vi "_PC_Daemon_System.vi"(7 "GetRef? ( F )":bool, 8 "error in (no error)":errorcluster) -> (0 "error out":errorcluster, 2 "Instrument Parmeter":T1)   [LabVIEW 2018]
uses:
  <vilib>/event_ctls.llb/eventvkey.ctl
  PublicSubVI/Class/QMH/QMH.lvclass
panel:
  in  "Config Tab":enum32{"RT Status", "Vacuum", "High Voltage"}(tab)
  out "Time":timestamp
  out "Wfm occupied":string
  out "Firmware Version":string="None"
  out "RT Resource":cluster{timestamp[], dbl[]}[](graph)
  out "Turbo speed":cluster{timestamp, "Double":dbl}[](graph)
  out "Turbo power":cluster{timestamp, "Double":dbl}[](graph)
  out "Pressure chart":cluster{timestamp, "Double":dbl}[](graph)
  out "Turbo pump status":string
  out "Voltage":cluster{timestamp[], dbl[]}[](graph)
  out "break":bool
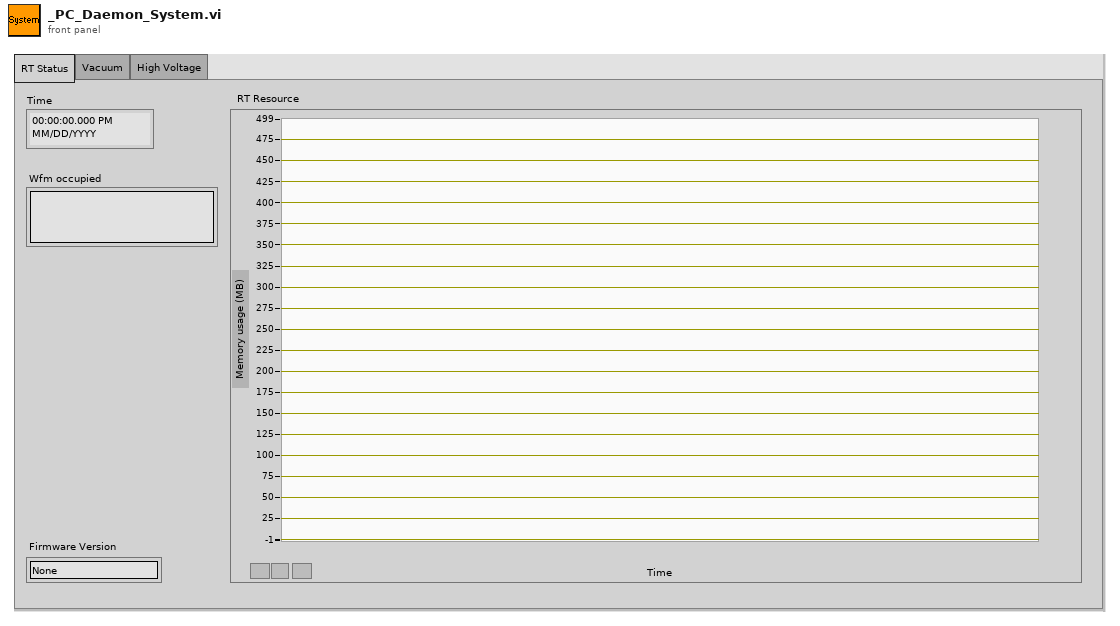
[diagram p1: front panel]
types:
  T1 = cluster{"Pressure chart":refnum<vi>, "Turbo pump status":refnum<vi>, "Turbo speed":refnum<vi>, "Turbo power":refnum<vi>, "RT Resource":refnum<vi>, "Pressure realtime":refnum<vi>, "Voltage":refnum<vi>, "Pressure string":refnum<vi>}
  T2 = typedef "eventvkey.ctl" = enum16{"ASCII", "Enter", "Return", "Shift", "Ctrl", "Alt", "Cmd", "Opt", "Caps", "NumLock", "Clear", "Break", "Up", "Down", "Left", "Right", "Insert", "Delete", "Home", "End", "PageUp", "PageDown", "Escape", "Help", "Pause", "ScrollLock", "F1", "F2", "F3", "F4", "F5", "F6", "F7", "F8", "F9", "F10", "F11", "F12", "F13", "F14", "F15", "F16", "F17", "F18", "F19", "F20", "F21", "F22", "F23", "F24", "Play", "VolumeUp", "VolumeDown", "Mute", "Two Byte Char"}
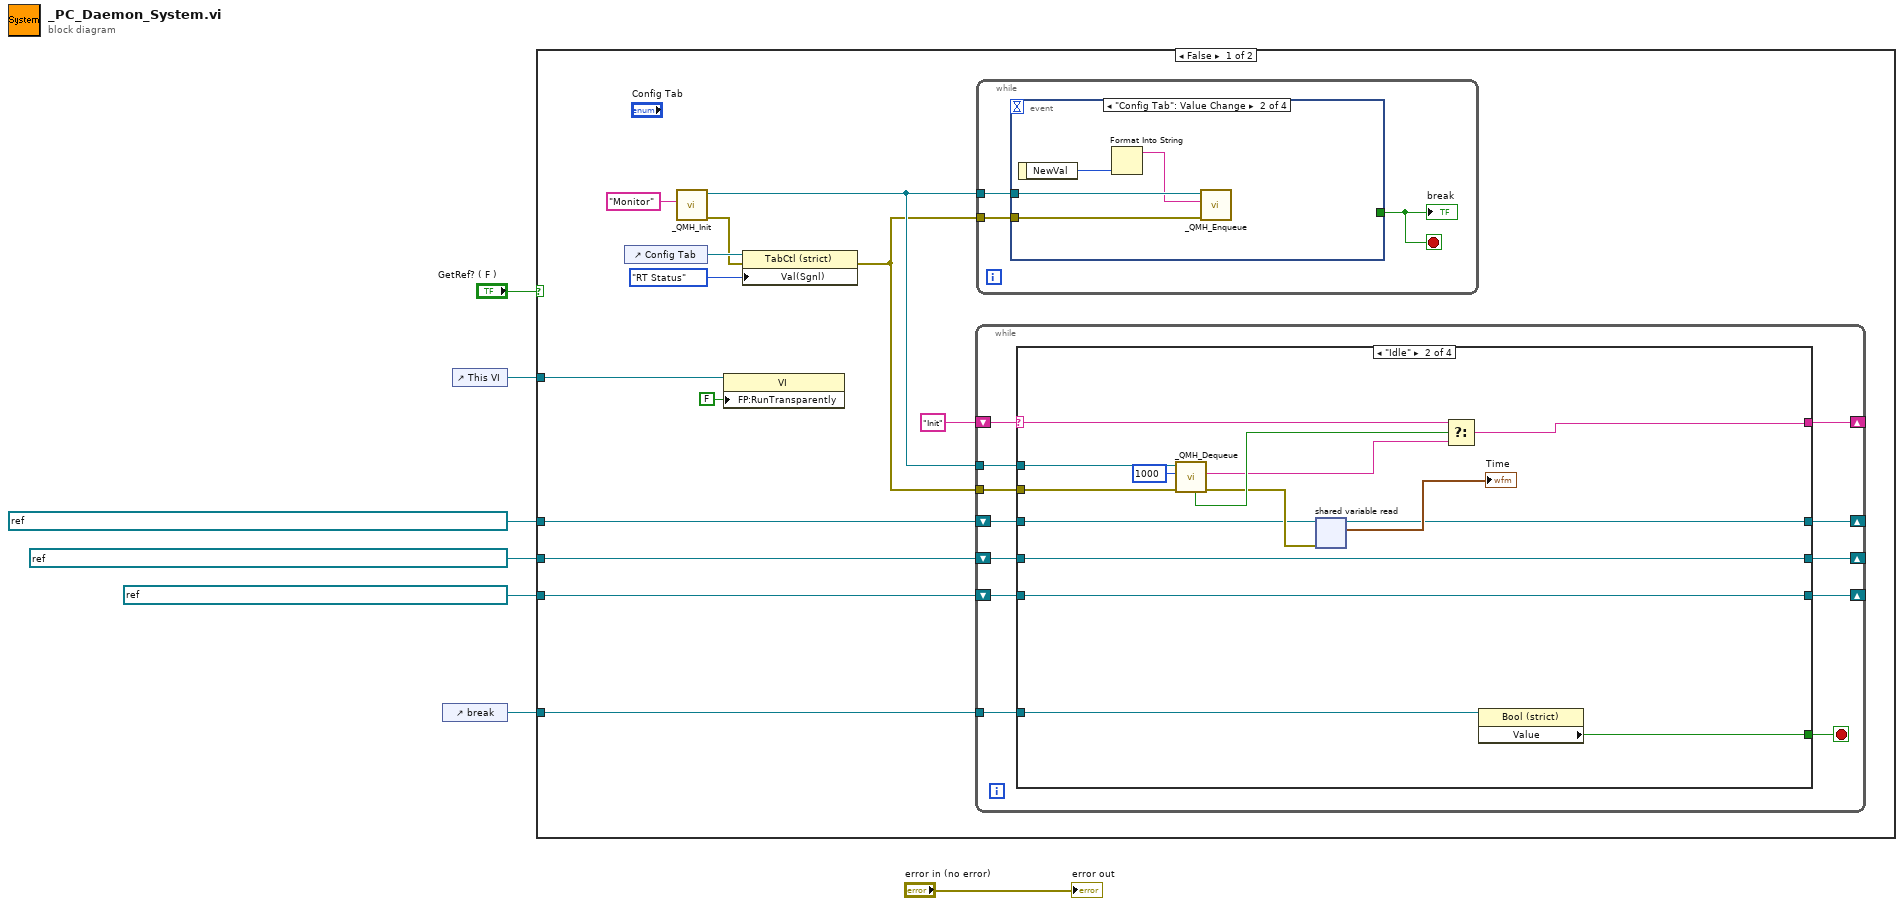
[diagram p0: block diagram]
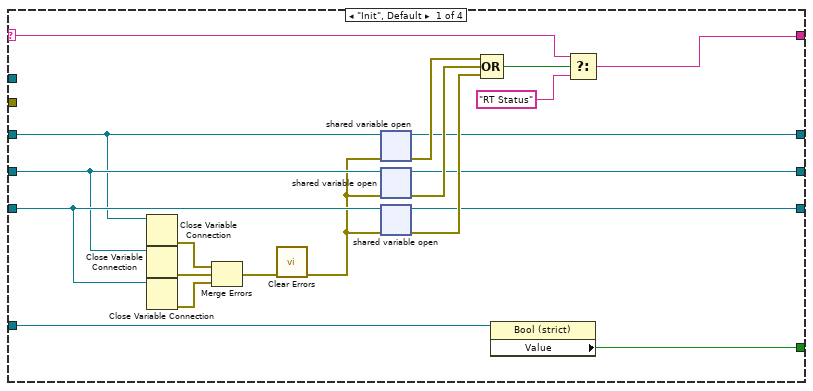
[diagram p2: hidden frame]
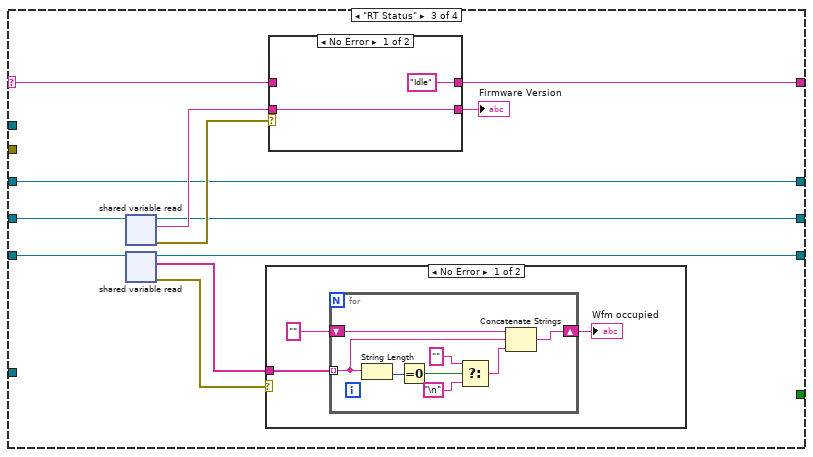
[diagram p3: hidden frame]
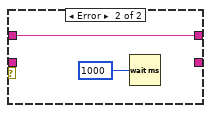
[diagram p4: hidden frame]
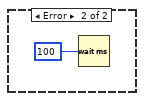
[diagram p5: hidden frame]
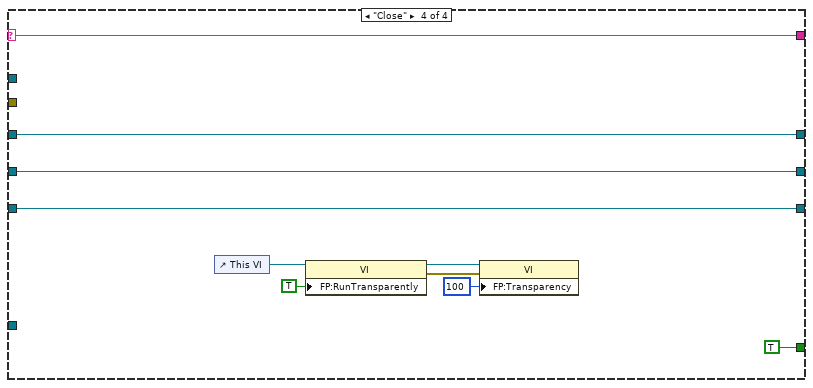
[diagram p6: hidden frame]
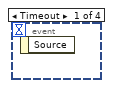
[diagram p7: hidden frame]
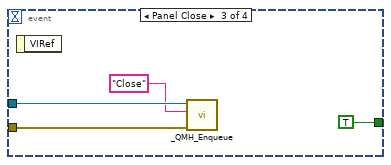
[diagram p8: hidden frame]
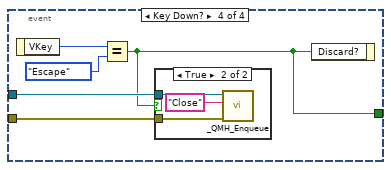
[diagram p9: hidden frame]
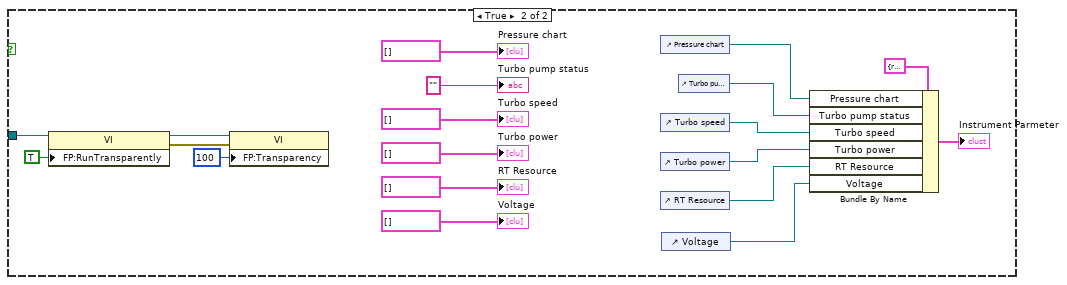
[diagram p11: hidden frame]
diagram:
  n1 = control-ref of="break"() -> (w1:refnum<vi>)
  n2 = control-ref of="This VI"() -> (w2:refnum<vi>)
  n3 = case shown="False" "GetRef? ( F )" {
    tunnel: refnum<k21> "ni.var.psp://NI-sbRIO/_RT_CtrlLoop_ResourcesMonitor_Variables/RT_SysTimeStamp" ("shared variable refnum in") -> [w14 _]
    tunnel: refnum<k21> "ni.var.psp://NI-sbRIO/_RT_CtrlLoop_ResourcesMonitor_Variables/SystemVersion" ("shared variable refnum in") -> [w13 _]
    tunnel: refnum<k21> "ni.var.psp://NI-sbRIO/_RT_Pub_Lib_SysVariables/OccupiedSizes" ("shared variable refnum in") -> [w12 _]
    tunnel: w2 -> [w10 w130]
    tunnel: w1 -> [w15 _]
    frame False {
      n4 = control-ref of="Config Tab"() -> (w17:refnum<vi>)
      n5 = call "_QMH_Init.vi"("name (unnamed)"="Monitor") -> ("error out"=w9:errorcluster, "QMH out"=w18:refnum<class "QMH.lvclass">)  [unwired: 9 in]
      n6 = property class="VI"(reference=w10, "FP:RunTransparently"=FALSE ("Front Panel Window:Run VI Transparently")) -> ()  [unwired: 1 in, 2 out]
      n7 = property class="TabCtl (strict)"(reference=w17, error in=w9, "Val(Sgnl)"=enum32{"RT Status", "Vacuum", "High Voltage"}."RT Status" ("Value")) -> (error out=w8:errorcluster)  [unwired: 1 out]
      n8 = while {
        shift-right: [w31] -> _
        shift-left: "Init" -> [w32]
        tunnel: w18 -> [w30]
        tunnel: w8 -> [w29]
        shift-right: [w24] -> _
        shift-left: w14 -> [w27]
        shift-right: [w23] -> _
        shift-left: w13 -> [w26]
        shift-right: [w22] -> _
        shift-left: w12 -> [w25]
        tunnel: w15 -> [w21]
        stop <- w28 stop-if-true
        n9 = case shown="\"Idle\"" w32 {
          selector: w32 -> [w40 w63 w79 w96]
          tunnel: [w38 w62 w78 w96] -> w31
          tunnel: w30 -> [_ w67 _ _]
          tunnel: w29 -> [_ w66 _ _]
          tunnel: [w33 w53 _ TRUE] -> w28
          tunnel: w27 -> [w47 w58 w70 w99]
          tunnel: w26 -> [w48 w56 w76 w98]
          tunnel: w25 -> [w49 w55 w75 w97]
          tunnel: [w37 w57 w70 w99] -> w24
          tunnel: [w36 w56 w69 w98] -> w23
          tunnel: [w35 w55 w68 w97] -> w22
          tunnel: w21 -> [w34 w54 _ _]
          frame "Init", Default {
            n10 = Close Variable Connection(11:w47) -> (0:w50:errorcluster)  [unwired: 1 in]
            n11 = Close Variable Connection(11:w48) -> (0:w51:errorcluster)  [unwired: 1 in]
            n12 = Close Variable Connection(11:w49) -> (0:w52:errorcluster)  [unwired: 1 in]
            n13 = Merge Errors(w50, w51, w52) -> (w46:errorcluster)
            n14 = call <vilib>:"Clear Errors.vi"("error in (no error)"=w46) -> ("error out"=w45:errorcluster)  [unwired: 5 in, 1 out]
            n15 = shared-variable-open(w47, w45) -> (w37:refnum<k21>, w44:errorcluster)
            n16 = shared-variable-open(w48, w45) -> (w36:refnum<k21>, w43:errorcluster)
            n17 = shared-variable-open(w49, w45) -> (w35:refnum<k21>, w42:errorcluster)
            n18 = Compound Arithmetic op=OR(w44, w43, w42) -> (w41:bool)
            n19 = property class="Bool (strict)"(reference=w34) -> ("Value"=w33:bool)  [unwired: 1 in, 2 out]
            n20 = Select(t=w40, s=w41, f="RT Status") -> (s? t:f=w38:string)
          }
          frame "Idle" {
            n21 = call "_QMH_Dequeue.vi"("error in (no error)"=w66, "timeout in ms (-1)"=1000, "QMH in"=w67) -> ("error out"=w59:errorcluster, "Msg"=w61:string, "timed out?"=w64:bool)  [unwired: 3 in, 3 out]
            n22 = shared-variable-read(w58, w59) -> (w57:refnum<k21>, →"Time":timestamp)  [unwired: 1 out]
            n23 = Select(t=w63, s=w64, f=w61) -> (s? t:f=w62:string)
            n24 = property class="Bool (strict)"(reference=w54) -> ("Value"=w53:bool)  [unwired: 1 in, 2 out]
          }
          frame "RT Status" {
            n25 = shared-variable-read(w76) -> (w69:refnum<k21>, w73:errorcluster, w74:string)  [unwired: 1 in]
            n26 = shared-variable-read(w75) -> (w68:refnum<k21>, w71:errorcluster, w72:string[])  [unwired: 1 in]
            n27 = case shown="No Error" w71 {
              tunnel: w72 -> [w85 _]
              frame No Error {
                n28 = for {
                  tunnel: w85 -> [w92] mode=indexing
                  shift-right: [w94] -> w84
                  shift-left: "" -> [w93]
                  n29 = String Length(string=w92) -> (length=w91:i32)
                  n30 = Equal To 0?(x=w91) -> (x = 0?=w90:bool)
                  n31 = Select(t="", s=w90, f="\n") -> (s? t:f=w87:string)
                  n32 = Concatenate Strings(w93, w92, w87) -> (w94:string)
                }
                "Wfm occupied" <- w84
              }
              frame Error {
                n33 = Wait (ms)(milliseconds to wait=u32 100) -> ()  [unwired: 1 out]
              }
            }
            n34 = case shown="No Error" w73 {
              tunnel: w74 -> [w80 _]
              tunnel: w79 -> [_ w82]
              tunnel: ["Idle" w82] -> w78
              tunnel: [w80 _] -> w77
              frame No Error {
              }
              frame Error {
                n35 = Wait (ms)(milliseconds to wait=u32 1000) -> ()  [unwired: 1 out]
              }
            }
            "Firmware Version" <- w77
          }
          frame "Close" {
            n36 = control-ref of="This VI"() -> (w104:refnum<vi>)
            n37 = property class="VI"(reference=w104, "FP:RunTransparently"=TRUE ("Front Panel Window:Run VI Transparently")) -> (reference out=w103:refnum<vi>, error out=w102:errorcluster)  [unwired: 1 in]
            n38 = property class="VI"(reference=w103, error in=w102, "FP:Transparency"=u8 100 ("Front Panel Window:Transparency")) -> ()  [unwired: 2 out]
          }
        }
      }
      n39 = while {
        tunnel: w18 -> [w108]
        tunnel: w8 -> [w107]
        stop <- w106 stop-if-true
        n40 = event shown="[1] \"Config Tab\": Value Change" {
          selector: _ -> [_ _ _ _]
          dyn-events: _ -> [_ _ _ _]
          timeout: _ -> [_ _ _ _]
          tunnel: w108 -> [_ w112 w116 w121]
          tunnel: w107 -> [_ w111 w115 w120]
          tunnel: [_ _ TRUE ("GetRef? ( F )") w117] -> w106
          event Timeout {
            n41 = event-data() -> ()  [unwired: 1 in, 1 out]
          }
          event "Config Tab": Value Change {
            n42 = event-data() -> ("NewVal"=w110:enum32{"RT Status", "Vacuum", "High Voltage"})  [unwired: 1 in]
            n43 = Format Into String(w110) -> (resulting string=w109:string)  [unwired: 3 in, 1 out]
            n44 = call "_QMH_Enqueue.vi"("error in (no error)"=w111, "Msg"=w109, "QMH in"=w112) -> ()  [unwired: 7 in, 2 out]
          }
          event Panel Close {
            n45 = event-data() -> ()  [unwired: 1 in, 1 out]
            n46 = call "_QMH_Enqueue.vi"("error in (no error)"=w115, "Msg"="Close", "QMH in"=w116) -> ()  [unwired: 7 in, 2 out]
          }
          event Key Down? {
            n47 = event-data() -> ("VKey"=w119:T2)  [unwired: 1 in]
            n48 = Equal?(x=w119, y=eventvkey."Escape" ("VKey")) -> (x = y?=w117:bool)
            n49 = case shown="True" w117 {
              tunnel: w121 -> [_ w124]
              tunnel: w120 -> [_ w123]
              frame False {
              }
              frame True {
                n50 = call "_QMH_Enqueue.vi"("error in (no error)"=w123, "Msg"="Close", "QMH in"=w124) -> ()  [unwired: 7 in, 2 out]
              }
            }
            n51 = event-data("Discard?"=w117) -> ()  [unwired: 1 in, 1 out]
          }
        }
        "break" <- w106
      }
    }
    frame True {
      n52 = property class="VI"(reference=w130, "FP:RunTransparently"=TRUE ("Front Panel Window:Run VI Transparently")) -> (reference out=w128:refnum<vi>, error out=w127:errorcluster)  [unwired: 1 in]
      n53 = property class="VI"(reference=w128, error in=w127, "FP:Transparency"=u8 100 ("Front Panel Window:Transparency")) -> ()  [unwired: 2 out]
      n54 = control-ref of="Pressure chart"() -> (w143:refnum<vi>)
      n55 = control-ref of="Turbo speed"() -> (w141:refnum<vi>)
      n56 = control-ref of="Turbo power"() -> (w140:refnum<vi>)
      n57 = control-ref of="RT Resource"() -> (w139:refnum<vi>)
      n58 = control-ref of="Voltage"() -> (w133:refnum<vi>)
      n59 = control-ref of="Turbo pump status"() -> (w142:refnum<vi>)
      n60 = Bundle By Name(cluster=T1 {"Pressure chart"=refnum, "Turbo pump status"=refnum, "Turbo speed"=refnum, "Turbo power"=refnum, "RT Resource"=refnum, "Pressure realtime"=refnum, "Voltage"=refnum, "Pressure string"=refnum} ("Instrument Parmeter"), "Pressure chart"=w143, "Turbo pump status"=w142, "Turbo speed"=w141, "Turbo power"=w140, "RT Resource"=w139, "Voltage"=w133) -> (→"Instrument Parmeter":T1)
      "Turbo power" <- cluster{timestamp, "Double":dbl}[] [] ("Turbo power")
      "Turbo speed" <- cluster{timestamp, "Double":dbl}[] [] ("Turbo speed")
      "Turbo pump status" <- "" ("Turbo pump status")
      "Pressure chart" <- cluster{timestamp, "Double":dbl}[] []
      "Voltage" <- cluster{timestamp[], dbl[]}[] [] ("Voltage")
      "RT Resource" <- cluster{timestamp[], dbl[]}[] [] ("RT Resource")
    }
  }
  "error out" <- "error in (no error)"
